vi "XIPIN_Image_Enhancement_8_0.vi"   [LabVIEW 2017]
doc: "The Xilinx Image Enhancement LogiCORE IP provides users with an easy-to-use IP block to reduce image noise and enhance the edges of objects in each picture. Two-dimensional filters are used to suppress noise while preserving and enhancing edges in the picture.\n------------------------------------\n<b>Need License</b> : Yes\n<b>Interface</b> : AXI4 AXI4-Stream"
uses:
  <vilib>/rvi/XilinxIP/XIPIN_XNode/niFpgaXIPIN.xnode
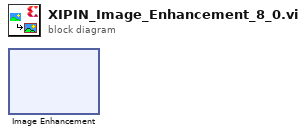
[diagram p0: block diagram]
diagram:
  n1 = xnode ("Image Enhancement")() -> ()
